vi "MAX-SP-RemoveResultChannel.vi"(8 "Error In":errorcluster, 11 "Device Ref in":T1 format="%.0x") -> (0 "Error Out":errorcluster, 3 "Device Ref Out":T1=18446744073709551615 format="%.0x")   [LabVIEW 2017, in "Waveform-Processing-Custom-Device Shared.lvlib" / "Max_SP.lvlib"]
doc: "This application Removes all of the Child \"Maximum\" output channels found when the \"Remove\" option is selected"
uses:
  Max_SP.lvlib
  <vilib>/NI Veristand/Custom Device API/Custom Device Item Ref.ctl
  Constants.vi
  <vilib>/NI Veristand/Custom Device API/Get Item Property (Dependent Node Pointer).vi
  System Explorer/Waveform-Processing-Custom-Device System Explorer.lvlib
  <vilib>/NI VeriStand/Custom Device API/Custom Device API.lvlib
  Waveform-Processing-Custom-Device Shared.lvlib
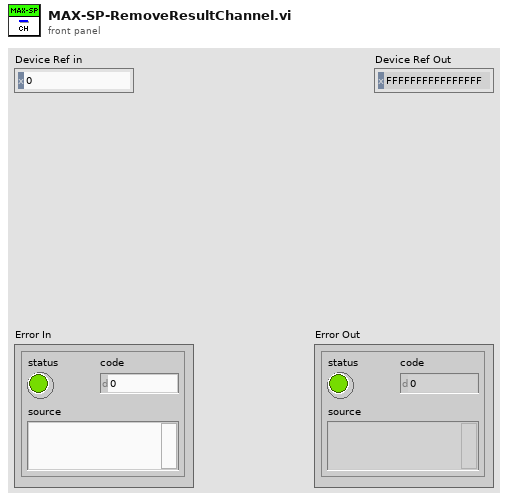
[diagram p1: front panel]
types:
  T1 = typedef "Custom Device API.lvlib/Custom Device Item Ref.ctl" = u64
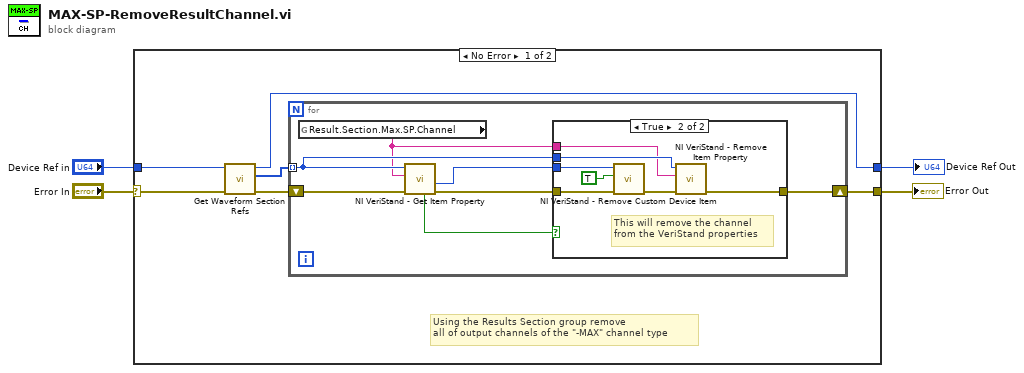
[diagram p0: block diagram]
diagram:
  n1 = case shown="No Error" "Error In" {
    selector: "Error In" -> [w9 w27]
    tunnel: "Device Ref in" -> [w10 w26]
    tunnel: [w7 w27] -> w2
    tunnel: [w5 w26] -> w1
    frame No Error {
      # "Using the Results Section group remove \nall of output channels of the \"-MAX\" channel type"
      n2 = call "Get Waveform Section Refs.vi"("Error in"=w9, "Device Ref in"=w10) -> ("Error out"=w8:errorcluster, "Result Section Refs"=w6:T1[], "Device Ref out"=w5:T1)  [unwired: 7 in]
      n3 = for {
        shift-right: [w14] -> w7
        shift-left: w8 -> [w15]
        tunnel: w6 -> [w13] mode=indexing
        n4 = global read "Constants.vi" "Result.Section.Max.SP.Channel"() -> (w12:string)
        n5 = call-poly <vilib>:"NI VeriStand - Get Item Property.vi"("error in (no error)"=w15, "Property Name"=w12, "Item Ref in"=w13) -> ("error out"=w16:errorcluster, "Dependent Node Ref"=w17:T1, "Found"=w11:bool)  [unwired: 5 in, 1 out]
        n6 = case shown="True" w11 {
          tunnel: w17 -> [_ w24]
          tunnel: w16 -> [w18 w23]
          tunnel: [w18 w21] -> w14
          tunnel: w13 -> [_ w20]
          tunnel: w12 -> [_ w19]
          frame False {
          }
          frame True {
            # "This will remove the channel \nfrom the VeriStand properties"
            n7 = call <vilib>:"NI VeriStand - Remove Custom Device Item.vi"("error in (no error)"=w23, "Force Delete (F)"=TRUE, "Item Ref in"=w24) -> ("error out"=w22:errorcluster)  [unwired: 7 in, 1 out]
            n8 = call <vilib>:"NI VeriStand - Remove Item Property.vi"("error in (no error)"=w22, "Property Name"=w19, "Item Ref in"=w20) -> ("error out"=w21:errorcluster)  [unwired: 6 in, 2 out]
          }
        }
      }
    }
    frame Error {
    }
  }
  "Error Out" <- w2
  "Device Ref Out" <- w1
